vi "PH_TKTDS-30xx.constructor.vi"(0 "name":string, 2 "data in":string, 5 "error in(no error)":errorcluster) -> (14 "i ref out":refnum<vi>, 16 "data out":string, 19 "error out":errorcluster)   [LabVIEW 2014, in "PH_TKTDS-30xx.lvlib"]
doc: "This is the constructor of a class.\n\nLicense Agreement for this software:\n\nCopyright (C)\nGesellschaft für Schwerionenforschung, GSI\nPlanckstr. 1\n64291 Darmstadt\nGermany\n\nContact: D.Beck@gsi.de \n\nThis program is free software; you can redistribute it and/or modify it under the terms of the \nGNU General Public License as published by the Free Software Foundation; either version 2 of \nthe license, or (at your option) any later version.\n\nThis program is distributed in the hope that it will be useful, but WITHOUT ANY WARRANTY; \nwithout even the implied warranty of MERCHANTABILITY or FITNESS FOR A PARTICULAR PURPOSE. See the GNU General License for more details (http://www.gnu.org).\n\nGesellschaft für Schwerionenforschung, GSI\nPlanckstr. 1, 64291 Darmstadt, Germany\nFor all questions and ideas contact: M.Richter@gsi.de, H.Brand@gsi.de or D.Beck@gsi.de.\nLast update: 16-JUN-2004"
uses:
  PH_TKTDS-30xx.lvlib
  CSCore/CSSystem/CSSystemLib/CSSystemLib.lvlib
  PH_PSDBWriter/PH_PSDBWriter.lvlib
  PH_Class/PH_Class.lvlib
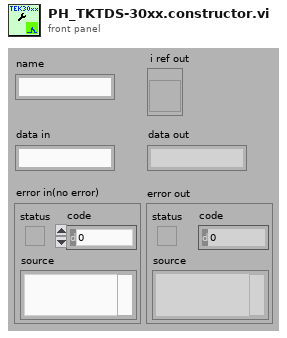
[diagram p1: front panel]
types:
  T1 = enum16{"SetAttribute", "GetAttribute", "CreateAttribute", "DestroyAttribute", "DestroyAllAtributes"}
  T2 = typedef "PH_TKTDS-30xx.lvlib/PH_TKTDS-30xx.i attribute.ctl" = cluster{"Default VISA Resource":string, "VISA Resource Name":refnum<visa-resource-name>, "Revision":cluster{"Instrument Driver":string, "Instrument Firmware":string}, "Selftest":cluster{"Result":u32, "Message":string}, "Channels":T3[], "Trigger Configuration":T4, "Acquisition Configuration":T5, "Fetched Waveforms":T6[], "GUI Refs":T7, "GUI Refs Channels":refnum<vi>[], "State":T8, "Error Message":string, "Allow Prdc Loop?":bool}
  T3 = typedef "PH_TKTDS-30xx.lvlib/PH_TKTDS-30xx.Channel Config.ctl" = cluster{"Channel Name":string, "Input Impedance":string, "Max Input Frequency":string, "Vertical Coupling":i32, "Channel Enabled":bool, "Probe Attenuation":dbl, "Vertical Range":dbl, "Vertical Offset":dbl}
  T4 = typedef "PH_TKTDS-30xx.lvlib/PH_TKTDS-30xx.Trigger Config.ctl" = cluster{"Source":string, "Slope":i32, "Level [V]":dbl}
  T5 = typedef "PH_TKTDS-30xx.lvlib/PH_TKTDS-30xx.Acquisition Config.ctl" = cluster{"Time base":dbl, "Record Length":u16, "Start Time":dbl, "Type":i32, "Continuous":bool}
  T6 = typedef "PH_TKTDS-30xx.lvlib/PH_TKTDS-30xx.fetched Waveform.ctl" = cluster{"Source":string, "Actual Points":u32, "Initial X":dbl, "X Increment":dbl, "Waveform Array":dbl[]}
  T7 = typedef "PH_TKTDS-30xx.lvlib/PH_TKTDS-30xx.GUI Refs.ctl" = cluster{"Trigger":refnum<vi>, "Acquisition":refnum<vi>, "Graph":refnum<vi>, "State":refnum<vi>, "Delete":refnum<vi>, "Channel to be positioned":refnum<vi>, "Postion":refnum<vi>, "Display Intensity":refnum<vi>, "VISA Resource":refnum<vi>}
  T8 = typedef "PH_StatusHandler.lvlib/PH_StatusHandler.Status.ctl" = i16
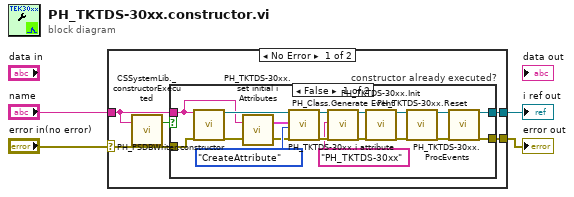
[diagram p0: block diagram]
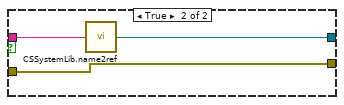
[diagram p2: hidden frame]
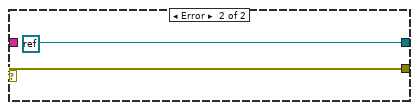
[diagram p3: hidden frame]
diagram:
  n1 = case shown="No Error" "error in(no error)" {
    selector: "error in(no error)" -> [w9 w31]
    tunnel: "name" -> [w8 _]
    tunnel: [w6 refnum<k0> refnum] -> w3
    tunnel: [w5 w31] -> w2
    frame No Error {
      n2 = call "CSSystemLib._constructorExecuted.vi"("name"=w8) -> ("constructor executed?"=w7:bool)  [unwired: 18 in]
      n3 = case "constructor already executed?" shown="False" w7 {
        tunnel: [w16 w29] -> w6
        tunnel: [w14 w28] -> w5
        tunnel: w9 -> [w27 w28]
        tunnel: w8 -> [w10 w30]
        frame False {
          n4 = call "PH_PSDBWriter.constructor.vi"("name"=w10, "error in"=w27) -> ("i ref out"=w11:refnum<vi>, "error out"=w13:errorcluster)  [unwired: 15 in, 1 out]
          n5 = call "PH_TKTDS-30xx.set initial i Attributes.vi"("error in"=w13, "Instance"=w10) -> ("error out"=w12:errorcluster, "i Attri"=w23:T2)
          n6 = call "PH_TKTDS-30xx.i attribute.vi"("VI Refnum"=w11, "CLASS.i attribute"=w23, "Action"=T1."CreateAttribute", "error in (no error)"=w12) -> ("VI Refnum out"=w22:refnum<vi>, "error out"=w20:errorcluster)  [unwired: 13 in, 1 out]
          n7 = call "PH_Class.Generate Event.vi"("i ref in"=w22, "Class"="PH_TKTDS-30xx", "error in (no error)"=w20) -> ("i ref out"=w21:refnum<vi>, "error out"=w19:errorcluster)  [unwired: 15 in]
          n8 = call "PH_TKTDS-30xx.Init.vi"("i ref in"=w21, "error in (no error)"=w19) -> ("i ref out"=w26:refnum<vi>, "error out"=w25:errorcluster)  [unwired: 16 in]
          n9 = call "PH_TKTDS-30xx.Reset.vi"("i ref in"=w26, "error IO"=w25) -> ("i ref out"=w17:refnum<vi>, "error out"=w15:errorcluster)  [unwired: 16 in]
          n10 = call "PH_TKTDS-30xx.ProcEvents.vi"("i ref in"=w17, "error in"=w15) -> ("i ref out"=w16:refnum<vi>, "error out"=w14:errorcluster)  [unwired: 16 in]
        }
        frame True {
          n11 = call "CSSystemLib.name2ref.vi"("name"=w30) -> ("obj refnum"=w29:refnum<vi>)
        }
      }
    }
    frame Error {
    }
  }
  "i ref out" <- w3
  "error out" <- w2
